vi "APC_9049_FilesPathFormation.vi"(3 "PostMortem":bool, 4 "ID":u32=6, 5 "TEST CODE":string) -> (0 "Full disk":bool, 1 "No disk":bool=TRUE, 2 "Files and paths":T1)   [LabVIEW 2020]
panel:
  out "CAS signals path":string
  out "free disk":dbl
  out "Saving path":string="/u/"
  out "CASfilePath":path
  out "CycleAVGfilePath":path
  out "AVGfilePath":path
  out "AVGfile":string
  out "CASfile":string
  out "CycleAVGfile":string
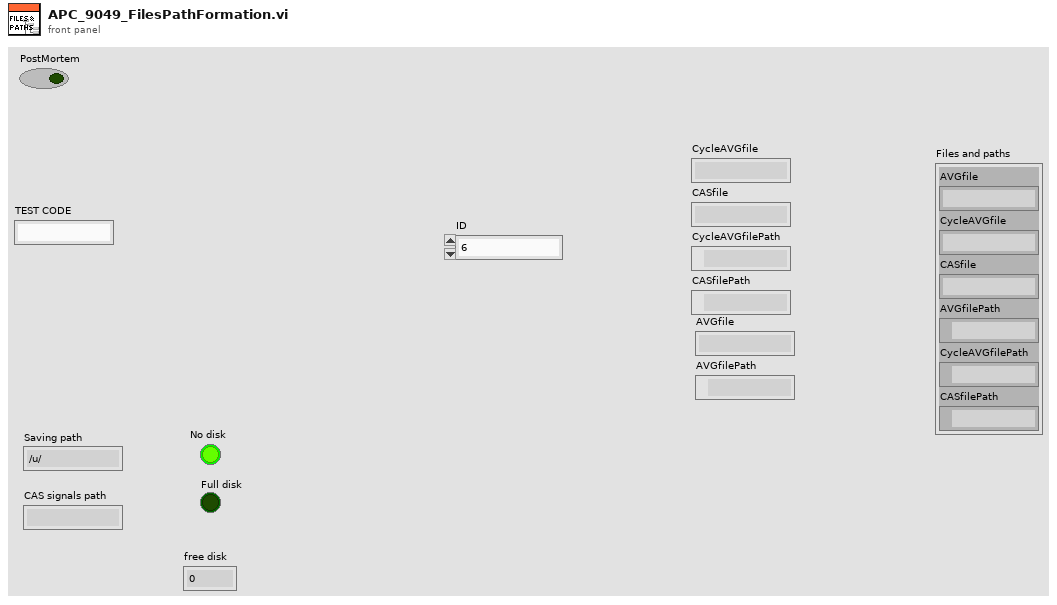
[diagram p1: front panel]
types:
  T1 = cluster{"AVGfile":string, "CycleAVGfile":string, "CASfile":string, "AVGfilePath":path, "CycleAVGfilePath":path, "CASfilePath":path}
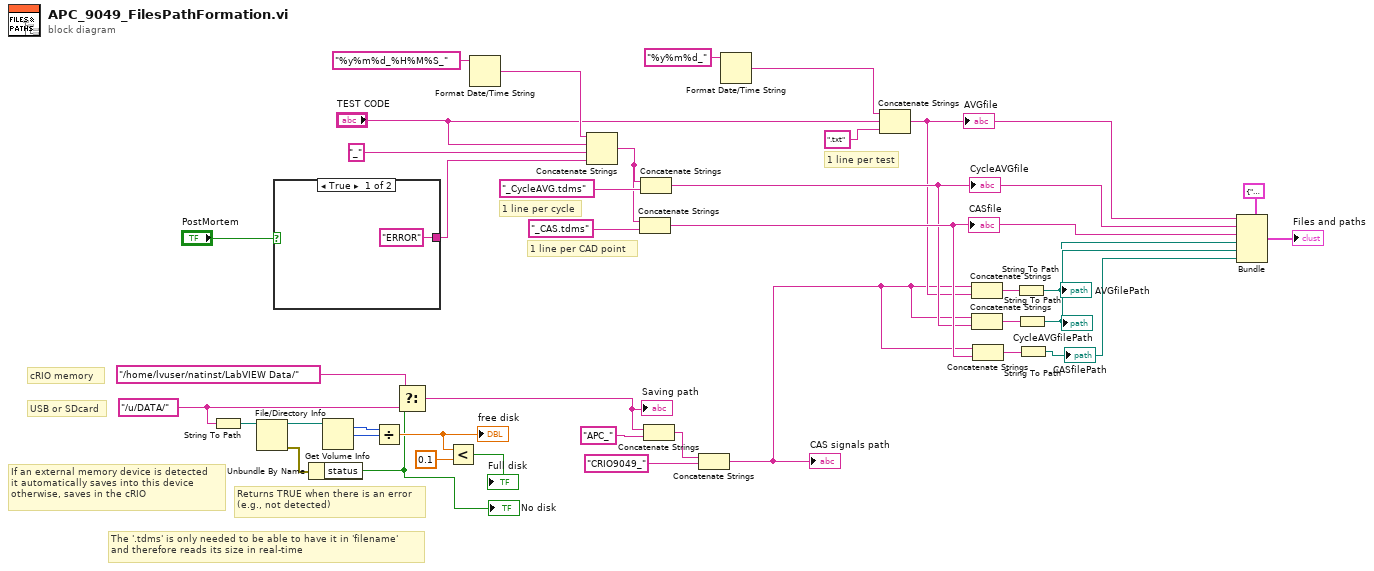
[diagram p0: block diagram]
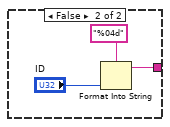
[diagram p2: hidden frame]
diagram:
  w4 = "/u/DATA/"
  # "If an external memory device is detected\nit automatically saves into this device\notherwise, saves in the cRIO"
  # "Returns TRUE when there is an error\n(e.g., not detected)"
  # "cRIO memory"
  # "USB or SDcard"
  # "The '.tdms' is only needed to be able to have it in 'filename'\nand therefore reads its size in real-time"
  # "1 line per CAD point"
  # "1 line per cycle"
  # "1 line per test"
  n1 = String To Path(string=w4) -> (path=w14:path)
  n2 = File/Directory Info(path=w14) -> (path out=w12:path, error out=w13:errorcluster)  [unwired: 1 in, 5 out]
  n3 = case shown="True" "PostMortem" {
    tunnel: ["ERROR" w42] -> w18
    frame True {
    }
    frame False {
      n4 = Format Into String(format string="%04d", "ID") -> (resulting string=w42:string)  [unwired: 2 in, 1 out]
    }
  }
  n5 = Unbundle By Name(w13) -> ("status"=w6:bool)
  "No disk" <- w6
  n6 = Get Volume Info(11:w12) -> (1:w10:i64, 2:w11:i64)  [unwired: 1 in, 4 out]
  n7 = Divide(x=w10, y=w11) -> (x/y=w9:dbl)
  "free disk" <- w9
  n8 = Select(t="/home/lvuser/natinst/LabVIEW Data/", s=w6, f=w4) -> (s? t:f=w3:string)
  "Saving path" <- w3
  n9 = Less?(x=w9, y=0.1) -> (x < y?=→"Full disk":bool)
  n10 = Format Date/Time String(time format string (%c)="%y%m%d_%H%M%S_") -> (date/time string=w37:string)  [unwired: 2 in]
  n11 = Concatenate Strings(w37, "TEST CODE", "_" ("string"), w18) -> (w30:string)
  n12 = Concatenate Strings(w30, "_CAS.tdms" ("string")) -> (w21:string)
  "CASfile" <- w21
  n13 = Concatenate Strings(w30, "_CycleAVG.tdms" ("string")) -> (w20:string)
  "CycleAVGfile" <- w20
  n14 = Concatenate Strings(w3, "APC_") -> (w15:string)
  n15 = Concatenate Strings(w15, "CRIO9049_") -> (w2:string)
  "CAS signals path" <- w2
  n16 = Format Date/Time String(time format string (%c)="%y%m%d_") -> (date/time string=w36:string)  [unwired: 2 in]
  n17 = Concatenate Strings(w36, "TEST CODE", ".txt" ("string")) -> (w19:string)
  "AVGfile" <- w19
  n18 = Concatenate Strings(w2, w19) -> (w29:string)
  n19 = Concatenate Strings(w2, w20) -> (w28:string)
  n20 = Concatenate Strings(w2, w21) -> (w27:string)
  n21 = String To Path(string=w29) -> (path=w22:path)
  "AVGfilePath" <- w22
  n22 = String To Path(string=w28) -> (path=w23:path)
  "CycleAVGfilePath" <- w23
  n23 = String To Path(string=w27) -> (path=w24:path)
  "CASfilePath" <- w24
  n24 = Bundle(cluster=T1 {"AVGfile"="", "CycleAVGfile"="", "CASfile"="", "AVGfilePath"=path "", "CycleAVGfilePath"=path "", "CASfilePath"=path ""} ("output cluster"), "AVGfile"=w19, "CycleAVGfile"=w20, "CASfile"=w21, "AVGfilePath"=w22, "CycleAVGfilePath"=w23, "CASfilePath"=w24) -> (→"Files and paths":T1)
